vi "Base_eleve.vi"() -> ()   [LabVIEW 2018]
uses:
  <vilib>/Instr/_visa.llb/VISA Configure Serial Port (Instr).vi
panel:
  out "Temperateur":dbl
  out "Chaîne":string
  in  "stop":bool
  in  "Nom de ressource VISA":refnum<visa-resource-name>
  # "1. Brancher la carte Arduino sur un port USB\n2. Choisir le port COM de la carte dans la liste déroulante \"Nom de ressource VISA\"\n3. Lancer le programme"
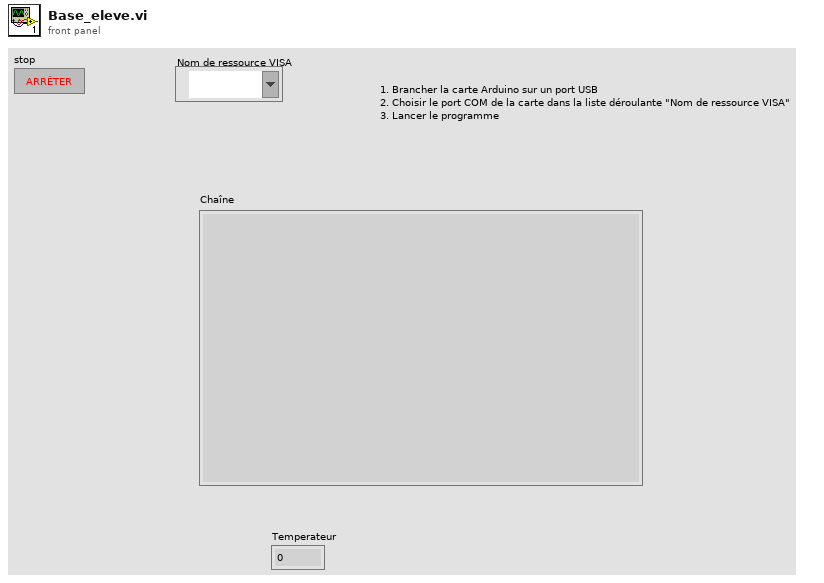
[diagram p1: front panel]
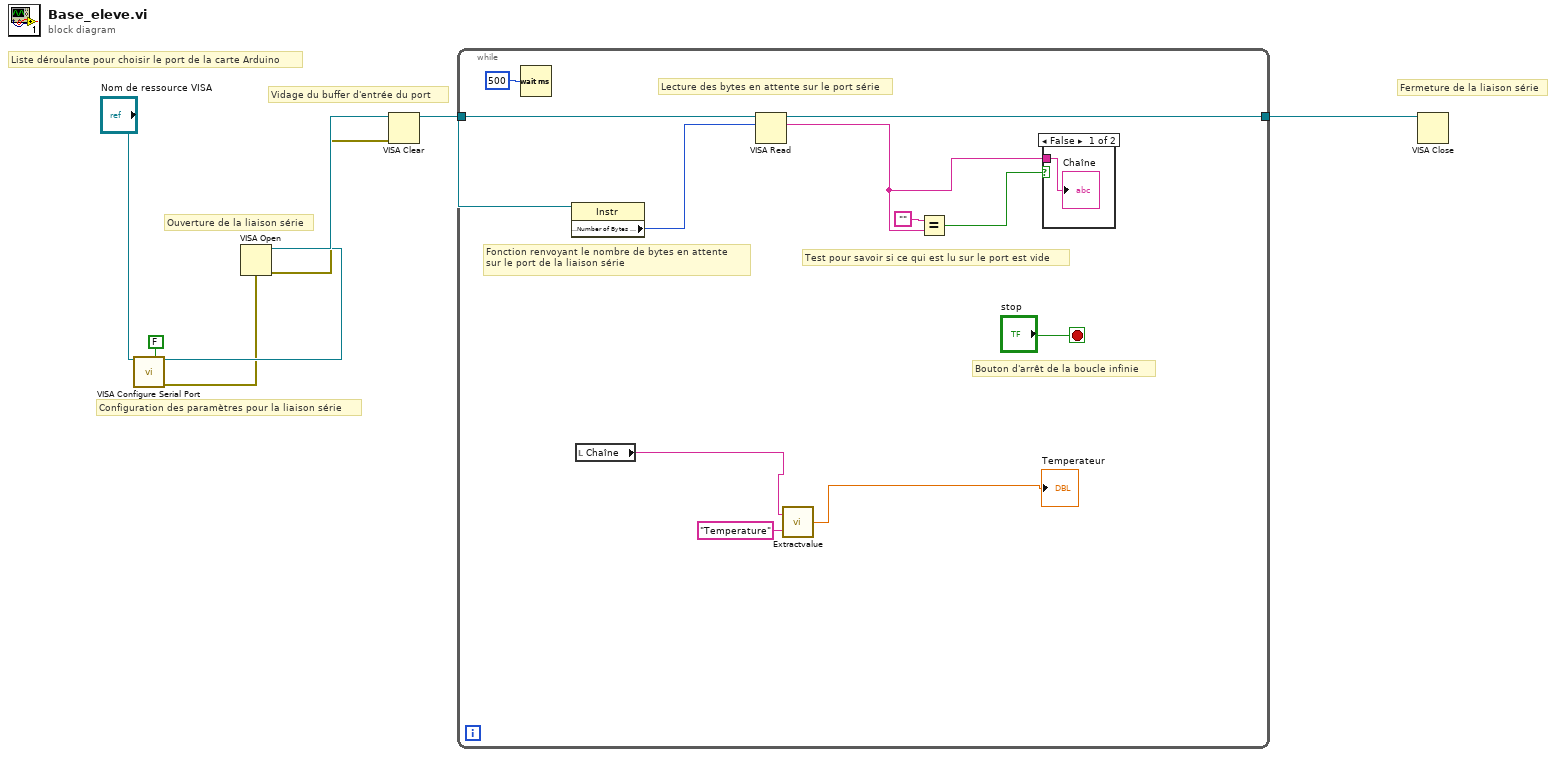
[diagram p0: block diagram]
diagram:
  # "Vidage du buffer d'entrée du port"
  # "Ouverture de la liaison série"
  # "Configuration des paramètres pour la liaison série"
  # "Liste déroulante pour choisir le port de la carte Arduino"
  # "Fermeture de la liaison série"
  n1 = call-poly "VISA Configure Serial Port"("VISA resource name"="Nom de ressource VISA", "Enable Termination\nChar (T)"=FALSE ("Enable Termination\nChar (T)")) -> ("VISA resource name out"=w5:refnum<visa-resource-name>, "error out"=w3:errorcluster)  [unwired: 12 in]
  n2 = VISA Open(error in (no error)=w3, VISA resource name=w5) -> (VISA resource name=w7:refnum<visa-resource-name>, error out=w2:errorcluster)  [unwired: 3 in]
  n3 = VISA Clear(VISA resource name=w7, error in (no error)=w2) -> (VISA resource name out=w6:refnum<visa-resource-name>)  [unwired: 1 out]
  n4 = while {
    tunnel: w6 -> [w18]
    tunnel: [w16] -> w1
    stop <- "stop" stop-if-true
    # "Lecture des bytes en attente sur le port série"
    # "Fonction renvoyant le nombre de bytes en attente\nsur le port de la liaison série"
    # "Test pour savoir si ce qui est lu sur le port est vide"
    # "Bouton d'arrêt de la boucle infinie"
    n5 = Wait (ms)(milliseconds to wait=u32 500 ("attente (ms)")) -> ()  [unwired: 1 out]
    n6 = property class="Instr"(reference=w18) -> ("Serial Settings:Number of Bytes at Serial Port"=w17:u32)  [unwired: 1 in, 2 out]
    n7 = local read "Chaîne"() -> (w11:string)
    n8 = VISA Read(VISA resource name=w18, byte count=w17) -> (VISA resource name out=w16:refnum<visa-resource-name>, read buffer=w12:string)  [unwired: 1 in, 2 out]
    n9 = call "Extractvalue.vi"("Mesure"="Temperature", "Chaîne"=w11) -> ("Value"=→"Temperateur":dbl)
    n10 = Equal?(x="", y=w12) -> (x = y?=w13:bool)
    n11 = case shown="False" w13 {
      tunnel: w12 -> [w20 _]
      frame False {
        "Chaîne" <- w20
      }
      frame True {
      }
    }
  }
  n12 = VISA Close(VISA resource name=w1) -> ()  [unwired: 1 in, 1 out]
